vi "update.vi"(8 "error in (no error)":errorcluster, 10 "Model in":refnum<class "Model.lvclass">, 11 "PerformOpenLoopScanState in":refnum<class "PerformOpenLoopScanState.lvclass">) -> (0 "error out":errorcluster, 2 "Model out":refnum<class "Model.lvclass">, 3 "PerformOpenLoopScanState out":refnum<class "PerformOpenLoopScanState.lvclass">)   [LabVIEW 2015, in "PerformOpenLoopScanState.lvclass"]
uses:
  PerformOpenLoopScanState.lvclass
  Model/Model/Model.lvclass
  Typedefs/StateSelector.ctl
  Typedefs/FAMTTypedefs.lvlib
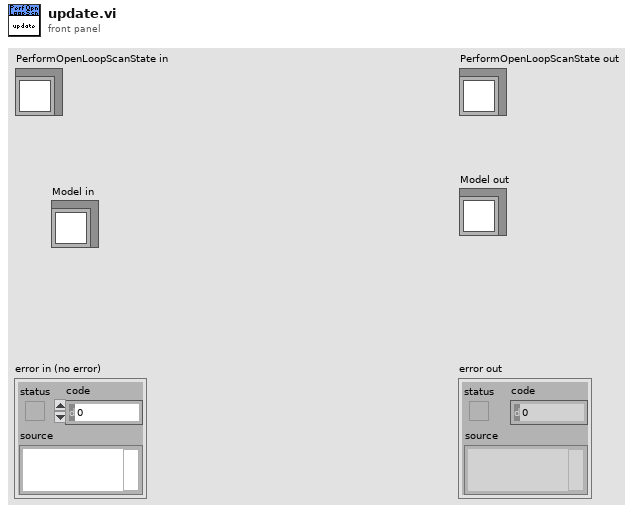
[diagram p1: front panel]
types:
  T1 = typedef "FAMTTypedefs.lvlib/StateSelector.ctl" = enum16{"OfflineState", "FaultState", "StandbyState", "DisabledState", "EnabledState", "WaitForUserInputState", "PerformOpenLoopScanState"}
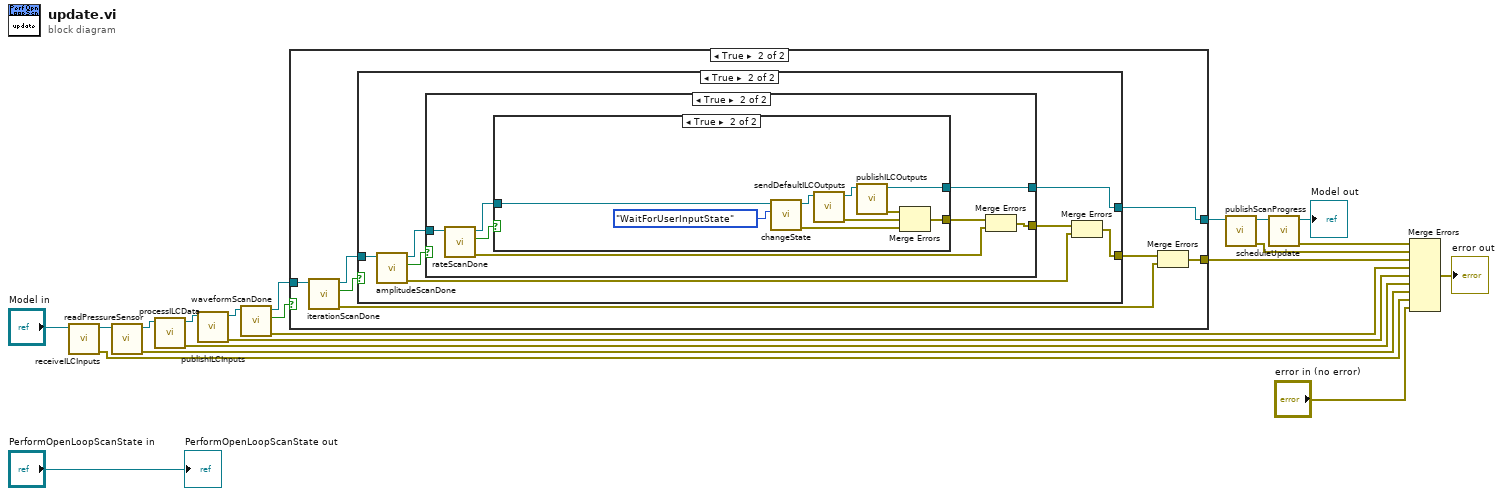
[diagram p0: block diagram]
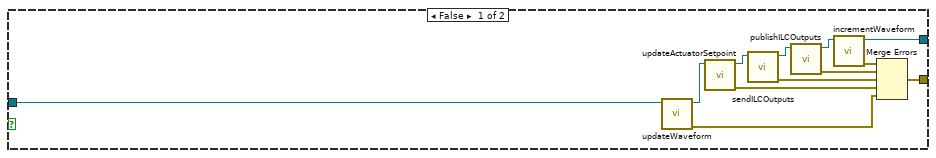
[diagram p2: hidden frame]
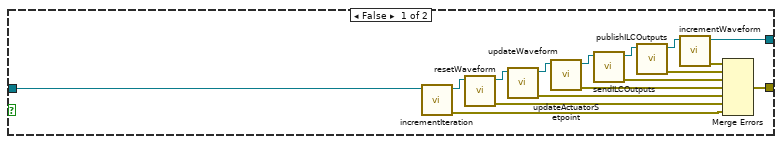
[diagram p3: hidden frame]
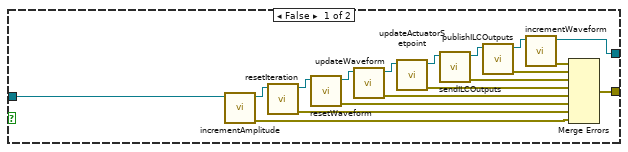
[diagram p4: hidden frame]
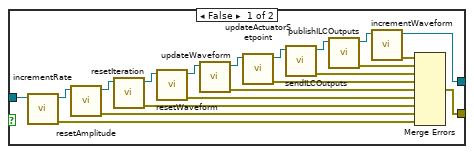
[diagram p5: hidden frame]
diagram:
  n1 = call "receiveILCInputs.vi"("Model in"="Model in") -> ("error out"=w17:errorcluster, "Model out"=w3:refnum<class "Model.lvclass">)  [unwired: 9 in]
  n2 = call "readPressureSensor.vi"("Model in"=w3) -> ("error out"=w1:errorcluster, "Model out"=w2:refnum<class "Model.lvclass">)  [unwired: 9 in]
  n3 = call "processILCData.vi"("Model in"=w2) -> ("error out"=w16:errorcluster, "Model out"=w21:refnum<class "Model.lvclass">)  [unwired: 9 in]
  n4 = call "publishILCInputs.vi"("Model in"=w21) -> ("error out"=w15:errorcluster, "Model out"=w7:refnum<class "Model.lvclass">)  [unwired: 9 in]
  n5 = call "waveformScanDone.vi"("Model in"=w7) -> ("error out"=w4:errorcluster, "Done?"=w9:bool, "Model out"=w8:refnum<class "Model.lvclass">)  [unwired: 8 in]
  n6 = case shown="True" w9 {
    tunnel: w8 -> [w23 w35]
    tunnel: [w26 w37] -> w5
    tunnel: [w25 w40] -> w6
    frame False {
      n7 = call "updateWaveform.vi"("Model in"=w23) -> ("error out"=w22:errorcluster, "Model out"=w24:refnum<class "Model.lvclass">)  [unwired: 9 in]
      n8 = call "updateActuatorSetpoint.vi"("Model in"=w24) -> ("error out"=w27:errorcluster, "Model out"=w33:refnum<class "Model.lvclass">)  [unwired: 9 in]
      n9 = call "sendILCOutputs.vi"("Model in"=w33) -> ("error out"=w28:errorcluster, "Model out"=w32:refnum<class "Model.lvclass">)  [unwired: 9 in]
      n10 = call "publishILCOutputs.vi"("Model in"=w32) -> ("error out"=w29:errorcluster, "Model out"=w31:refnum<class "Model.lvclass">)  [unwired: 9 in]
      n11 = call "incrementWaveform.vi"("Model in"=w31) -> ("error out"=w30:errorcluster, "Model out"=w25:refnum<class "Model.lvclass">)  [unwired: 9 in]
      n12 = Merge Errors(w30, w29, w28, w27, w22) -> (w26:errorcluster)
    }
    frame True {
      n13 = call "iterationScanDone.vi"("Model in"=w35) -> ("error out"=w39:errorcluster, "Done?"=w36:bool, "Model out"=w34:refnum<class "Model.lvclass">)  [unwired: 8 in]
      n14 = case shown="True" w36 {
        tunnel: w34 -> [w41 w61]
        tunnel: [w42 w60] -> w38
        tunnel: [w43 w57] -> w40
        frame False {
          n15 = call "incrementIteration.vi"("Model in"=w41) -> ("error out"=w44:errorcluster, "Model out"=w46:refnum<class "Model.lvclass">)  [unwired: 9 in]
          n16 = call "resetWaveform.vi"("Model in"=w46) -> ("error out"=w45:errorcluster, "Model out"=w47:refnum<class "Model.lvclass">)  [unwired: 9 in]
          n17 = call "updateWaveform.vi"("Model in"=w47) -> ("error out"=w48:errorcluster, "Model out"=w49:refnum<class "Model.lvclass">)  [unwired: 9 in]
          n18 = call "updateActuatorSetpoint.vi"("Model in"=w49) -> ("error out"=w50:errorcluster, "Model out"=w56:refnum<class "Model.lvclass">)  [unwired: 9 in]
          n19 = call "sendILCOutputs.vi"("Model in"=w56) -> ("error out"=w51:errorcluster, "Model out"=w55:refnum<class "Model.lvclass">)  [unwired: 9 in]
          n20 = call "publishILCOutputs.vi"("Model in"=w55) -> ("error out"=w52:errorcluster, "Model out"=w54:refnum<class "Model.lvclass">)  [unwired: 9 in]
          n21 = call "incrementWaveform.vi"("Model in"=w54) -> ("error out"=w53:errorcluster, "Model out"=w43:refnum<class "Model.lvclass">)  [unwired: 9 in]
          n22 = Merge Errors(w53, w52, w51, w50, w48, w45, w44) -> (w42:errorcluster)
        }
        frame True {
          n23 = call "amplitudeScanDone.vi"("Model in"=w61) -> ("error out"=w58:errorcluster, "Done?"=w63:bool, "Model out"=w62:refnum<class "Model.lvclass">)  [unwired: 8 in]
          n24 = case shown="True" w63 {
            tunnel: w62 -> [w81 w87]
            tunnel: [w71 w85] -> w59
            tunnel: [w70 w82] -> w57
            frame False {
              n25 = call "incrementAmplitude.vi"("Model in"=w81) -> ("error out"=w72:errorcluster, "Model out"=w66:refnum<class "Model.lvclass">)  [unwired: 9 in]
              n26 = call "resetIteration.vi"("Model in"=w66) -> ("error out"=w64:errorcluster, "Model out"=w65:refnum<class "Model.lvclass">)  [unwired: 9 in]
              n27 = call "resetWaveform.vi"("Model in"=w65) -> ("error out"=w73:errorcluster, "Model out"=w69:refnum<class "Model.lvclass">)  [unwired: 9 in]
              n28 = call "updateWaveform.vi"("Model in"=w69) -> ("error out"=w67:errorcluster, "Model out"=w68:refnum<class "Model.lvclass">)  [unwired: 9 in]
              n29 = call "updateActuatorSetpoint.vi"("Model in"=w68) -> ("error out"=w74:errorcluster, "Model out"=w80:refnum<class "Model.lvclass">)  [unwired: 9 in]
              n30 = call "sendILCOutputs.vi"("Model in"=w80) -> ("error out"=w75:errorcluster, "Model out"=w79:refnum<class "Model.lvclass">)  [unwired: 9 in]
              n31 = call "publishILCOutputs.vi"("Model in"=w79) -> ("error out"=w76:errorcluster, "Model out"=w78:refnum<class "Model.lvclass">)  [unwired: 9 in]
              n32 = call "incrementWaveform.vi"("Model in"=w78) -> ("error out"=w77:errorcluster, "Model out"=w70:refnum<class "Model.lvclass">)  [unwired: 9 in]
              n33 = Merge Errors(w77, w76, w75, w74, w67, w73, w64, w72) -> (w71:errorcluster)
            }
            frame True {
              n34 = call "rateScanDone.vi"("Model in"=w87) -> ("error out"=w83:errorcluster, "Done?"=w88:bool, "Model out"=w86:refnum<class "Model.lvclass">)  [unwired: 8 in]
              n35 = case shown="True" w88 {
                tunnel: w86 -> [w105 w116]
                tunnel: [w96 w110] -> w84
                tunnel: [w95 w109] -> w82
                frame False {
                  n36 = call "incrementRate.vi"("Model in"=w105) -> ("error out"=w97:errorcluster, "Model out"=w104:refnum<class "Model.lvclass">)  [unwired: 9 in]
                  n37 = call "resetAmplitude.vi"("Model in"=w104) -> ("error out"=w98:errorcluster, "Model out"=w91:refnum<class "Model.lvclass">)  [unwired: 9 in]
                  n38 = call "resetIteration.vi"("Model in"=w91) -> ("error out"=w89:errorcluster, "Model out"=w90:refnum<class "Model.lvclass">)  [unwired: 9 in]
                  n39 = call "resetWaveform.vi"("Model in"=w90) -> ("error out"=w99:errorcluster, "Model out"=w94:refnum<class "Model.lvclass">)  [unwired: 9 in]
                  n40 = call "updateWaveform.vi"("Model in"=w94) -> ("error out"=w92:errorcluster, "Model out"=w93:refnum<class "Model.lvclass">)  [unwired: 9 in]
                  n41 = call "updateActuatorSetpoint.vi"("Model in"=w93) -> ("error out"=w100:errorcluster, "Model out"=w108:refnum<class "Model.lvclass">)  [unwired: 9 in]
                  n42 = call "sendILCOutputs.vi"("Model in"=w108) -> ("error out"=w101:errorcluster, "Model out"=w107:refnum<class "Model.lvclass">)  [unwired: 9 in]
                  n43 = call "publishILCOutputs.vi"("Model in"=w107) -> ("error out"=w102:errorcluster, "Model out"=w106:refnum<class "Model.lvclass">)  [unwired: 9 in]
                  n44 = call "incrementWaveform.vi"("Model in"=w106) -> ("error out"=w103:errorcluster, "Model out"=w95:refnum<class "Model.lvclass">)  [unwired: 9 in]
                  n45 = Merge Errors(w103, w102, w101, w100, w92, w99, w89, w98, w97) -> (w96:errorcluster)
                }
                frame True {
                  n46 = call "changeState.vi"("State:"=StateSelector."WaitForUserInputState", "Model in"=w116) -> ("error out"=w111:errorcluster, "Model out"=w115:refnum<class "Model.lvclass">)  [unwired: 8 in]
                  n47 = call "sendDefaultILCOutputs.vi"("Model in"=w115) -> ("error out"=w112:errorcluster, "Model out"=w114:refnum<class "Model.lvclass">)  [unwired: 9 in]
                  n48 = call "publishILCOutputs.vi"("Model in"=w114) -> ("error out"=w113:errorcluster, "Model out"=w109:refnum<class "Model.lvclass">)  [unwired: 9 in]
                  n49 = Merge Errors(w113, w112, w111) -> (w110:errorcluster)
                }
              }
              n50 = Merge Errors(w84, w83) -> (w85:errorcluster)
            }
          }
          n51 = Merge Errors(w59, w58) -> (w60:errorcluster)
        }
      }
      n52 = Merge Errors(w38, w39) -> (w37:errorcluster)
    }
  }
  n53 = call "publishScanProgress.vi"("Model in"=w6) -> ("error out"=w11:errorcluster, "Model out"=w10:refnum<class "Model.lvclass">)  [unwired: 9 in]
  n54 = call "scheduleUpdate.vi"("Model in"=w10) -> ("error out"=w13:errorcluster, "Model out"=→"Model out":refnum<class "Model.lvclass">)  [unwired: 9 in]
  n55 = Merge Errors(w13, w11, w5, w4, w15, w16, w1, w17, "error in (no error)") -> (→"error out":errorcluster)
  "PerformOpenLoopScanState out" <- "PerformOpenLoopScanState in"
